vi "实验结果汇总子VI.vi"(5 "reference in":refnum<vi>) -> ()   [LabVIEW 2013]
uses:
  GlobleVar/IndentLevel.vi
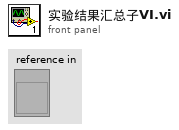
[diagram p1: front panel]
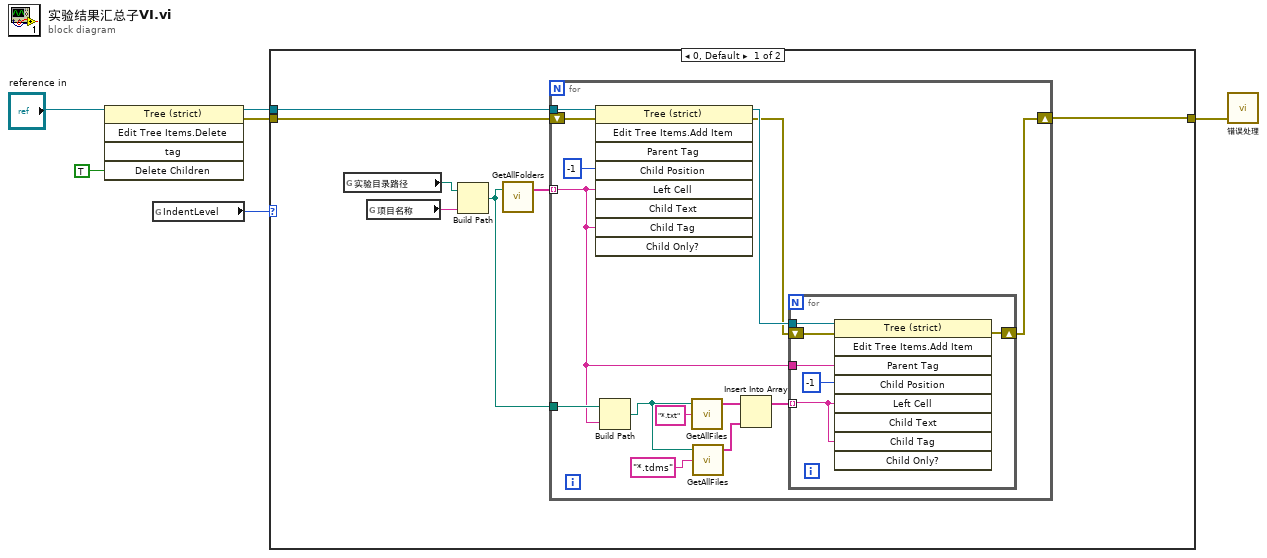
[diagram p0: block diagram]
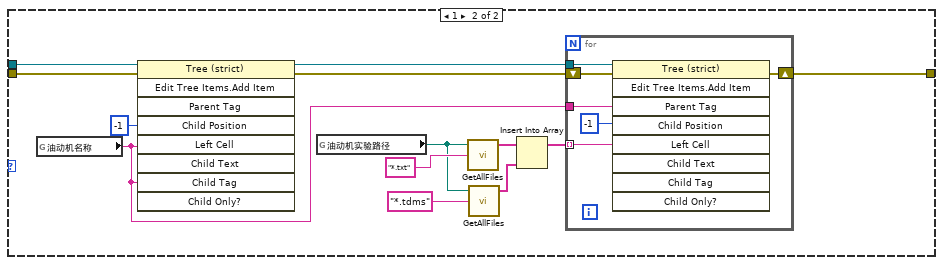
[diagram p2: hidden frame]
diagram:
  n1 = invoke class="Tree (strict)" method="Edit Tree Items.Delete"(reference="reference in", "Delete Children"=TRUE) -> (reference out=w4:refnum<vi>, error out=w2:errorcluster)  [unwired: 3 in, 3 out]
  n2 = global read "IndentLevel.vi" "IndentLevel"() -> (w5:i32)
  n3 = case shown="0, Default" w5 {
    tunnel: w4 -> [w9 w46]
    tunnel: w2 -> [w8 w36]
    tunnel: [w7 w34] -> w1
    frame 0, Default {
      n4 = global read "实验目录路径.vi" "实验目录路径"() -> (w11:path)
      n5 = global read "项目名称.vi" "项目名称"() -> (w12:string)
      n6 = Build Path(base path=w11, name or relative path=w12) -> (appended path=w10:path)
      n7 = call "GetAllFolders.vi"("FolderPath"=w10) -> ("Folders"=w13:string[])  [unwired: 1 in, 1 out]
      n8 = for {
        tunnel: w13 -> [w25] mode=indexing
        tunnel: w10 -> [w26]
        tunnel: w9 -> [w23]
        shift-right: [w14] -> w7
        shift-left: w8 -> [w16]
        n9 = invoke class="Tree (strict)" method="Edit Tree Items.Add Item"(reference=w23, error in=w16, "Child Position"=-1, "Left Cell"=w25, "Child Tag"=w25) -> (reference out=w24:refnum<vi>, error out=w15:errorcluster)  [unwired: 4 in, 7 out]
        n10 = Build Path(base path=w26, name or relative path=w25) -> (appended path=w20:path)
        n11 = call "GetAllFiles.vi"("Pattern"="*.txt", "FolderPath"=w20) -> ("Files"=w22:string[])  [unwired: 2 in, 1 out]
        n12 = call "GetAllFiles.vi"("Pattern"="*.tdms", "FolderPath"=w20) -> ("Files"=w21:string[])  [unwired: 2 in, 1 out]
        n13 = Insert Into Array(array=w22, new element=w21) -> (w19:string[])  [unwired: 1 in]
        n14 = for {
          tunnel: w19 -> [w33] mode=indexing
          tunnel: w25 -> [w31]
          tunnel: w24 -> [w30]
          shift-right: [w28] -> w14
          shift-left: w15 -> [w29]
          n15 = invoke class="Tree (strict)" method="Edit Tree Items.Add Item"(reference=w30, error in=w29, "Parent Tag"=w31, "Child Position"=-1, "Left Cell"=w33, "Child Tag"=w33) -> (error out=w28:errorcluster)  [unwired: 3 in, 8 out]
        }
      }
    }
    frame 1 {
      n16 = global read "油动机名称.vi" "油动机名称"() -> (w44:string)
      n17 = invoke class="Tree (strict)" method="Edit Tree Items.Add Item"(reference=w46, error in=w36, "Child Position"=-1, "Left Cell"=w44, "Child Tag"=w44) -> (reference out=w45:refnum<vi>, error out=w35:errorcluster)  [unwired: 4 in, 7 out]
      n18 = global read "油动机实验路径.vi" "油动机实验路径"() -> (w41:path)
      n19 = call "GetAllFiles.vi"("Pattern"="*.txt", "FolderPath"=w41) -> ("Files"=w38:string[])  [unwired: 2 in, 1 out]
      n20 = call "GetAllFiles.vi"("Pattern"="*.tdms", "FolderPath"=w41) -> ("Files"=w37:string[])  [unwired: 2 in, 1 out]
      n21 = Insert Into Array(array=w38, new element=w37) -> (w39:string[])  [unwired: 1 in]
      n22 = for {
        tunnel: w45 -> [w51]
        tunnel: w44 -> [w50]
        tunnel: w39 -> [w49] mode=indexing
        shift-right: [w47] -> w34
        shift-left: w35 -> [w48]
        n23 = invoke class="Tree (strict)" method="Edit Tree Items.Add Item"(reference=w51, error in=w48, "Parent Tag"=w50, "Child Position"=-1, "Left Cell"=w49) -> (error out=w47:errorcluster)  [unwired: 4 in, 8 out]
      }
    }
  }
  n24 = call "错误处理.vi"("error in (no error)"=w1) -> ()  [unwired: 2 in]
